vi "Double from Pointer.vi"(4 "Type":dbl format="%.2f", 5 "error in (no error)":errorcluster, 8 "Pointer":i32) -> (0 "error out":errorcluster, 2 "data":dbl format="%.2f", 3 "Duplicate Pointer":i32)   [LabVIEW 2011]
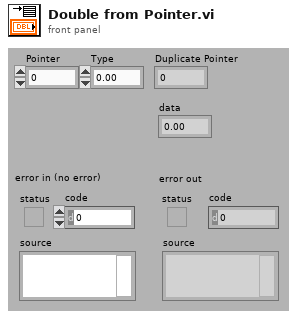
[diagram p1: front panel]
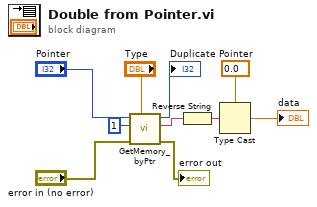
[diagram p0: block diagram]
diagram:
  n1 = call "GetMemory_byPtr.vi"("Data Type"="Type", "error in (no error)"="error in (no error)", "Data Size(1)"=1, "Pointer"="Pointer") -> ("error out"=→"error out":errorcluster, "data"=w7:string, "Duplicate Pointer"=→"Duplicate Pointer":i32)  [unwired: 2 out]
  n2 = Reverse String(1:w7) -> (0:w6:string)
  n3 = Type Cast(type=0.0, x=w6) -> (*(type *) &x=→"data":dbl)
